vi "callC.vi"(8 "error in (no error)":errorcluster, 9 "constant command line":T1={"Red ball"={"R max"=255, "R min"=91, "G max"=80, "B max"=130, "B min"=0, "G min"=0}, "Yellow ball"={"R max"=255, "R min"=170, "G max"=255, "B max"=175, "B min"=0, "G min"=176}, "White ball"={"R max"=255, "R min"=100, "G max"=255, "B max"=250, "B min"=150, "G min"=150}, "Blue BG"={"R max"=62, "R min"=39, "G max"=116, "B max"=255, "B min"=202, "G min"=91}, "Ball diameter"=13}, 10 "billard rect":T2, 11 "Array":u32[][](array[numeric])) -> (0 "error out":errorcluster, 1 "White":cluster{"X":string, "Y":string}, 2 "Yellow":cluster{"X":string, "Y":string}, 3 "Red":cluster{"X":string, "Y":string}, 4 "standard error":string, 5 "standard output":string)   [LabVIEW 2021]
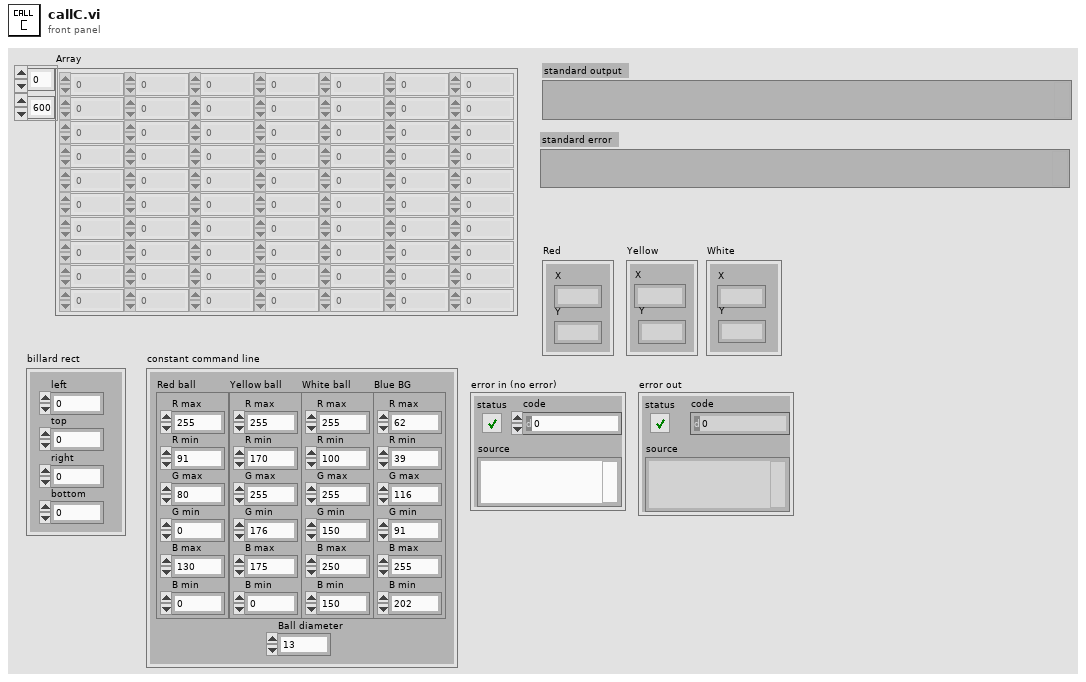
[diagram p1: front panel]
types:
  T1 = cluster{"Red ball":cluster{"R max":u8, "R min":u8, "G max":u8, "B max":u8, "B min":u8, "G min":u8}, "Yellow ball":cluster{"R max":u8, "R min":u8, "G max":u8, "B max":u8, "B min":u8, "G min":u8}, "White ball":cluster{"R max":u8, "R min":u8, "G max":u8, "B max":u8, "B min":u8, "G min":u8}, "Blue BG":cluster{"R max":u8, "R min":u8, "G max":u8, "B max":u8, "B min":u8, "G min":u8}, "Ball diameter":i32}
  T2 = cluster{"left":i32, "top":i32, "right":i32, "bottom":i32}
  T3 = enum16{"open", "replace", "create", "open or create", "replace or create", "replace or create with confirmation"}
  T4 = enum16{"big-endian, network order", "native, host order", "little-endian"}
  T5 = cluster{"result string":string, "result string":string}
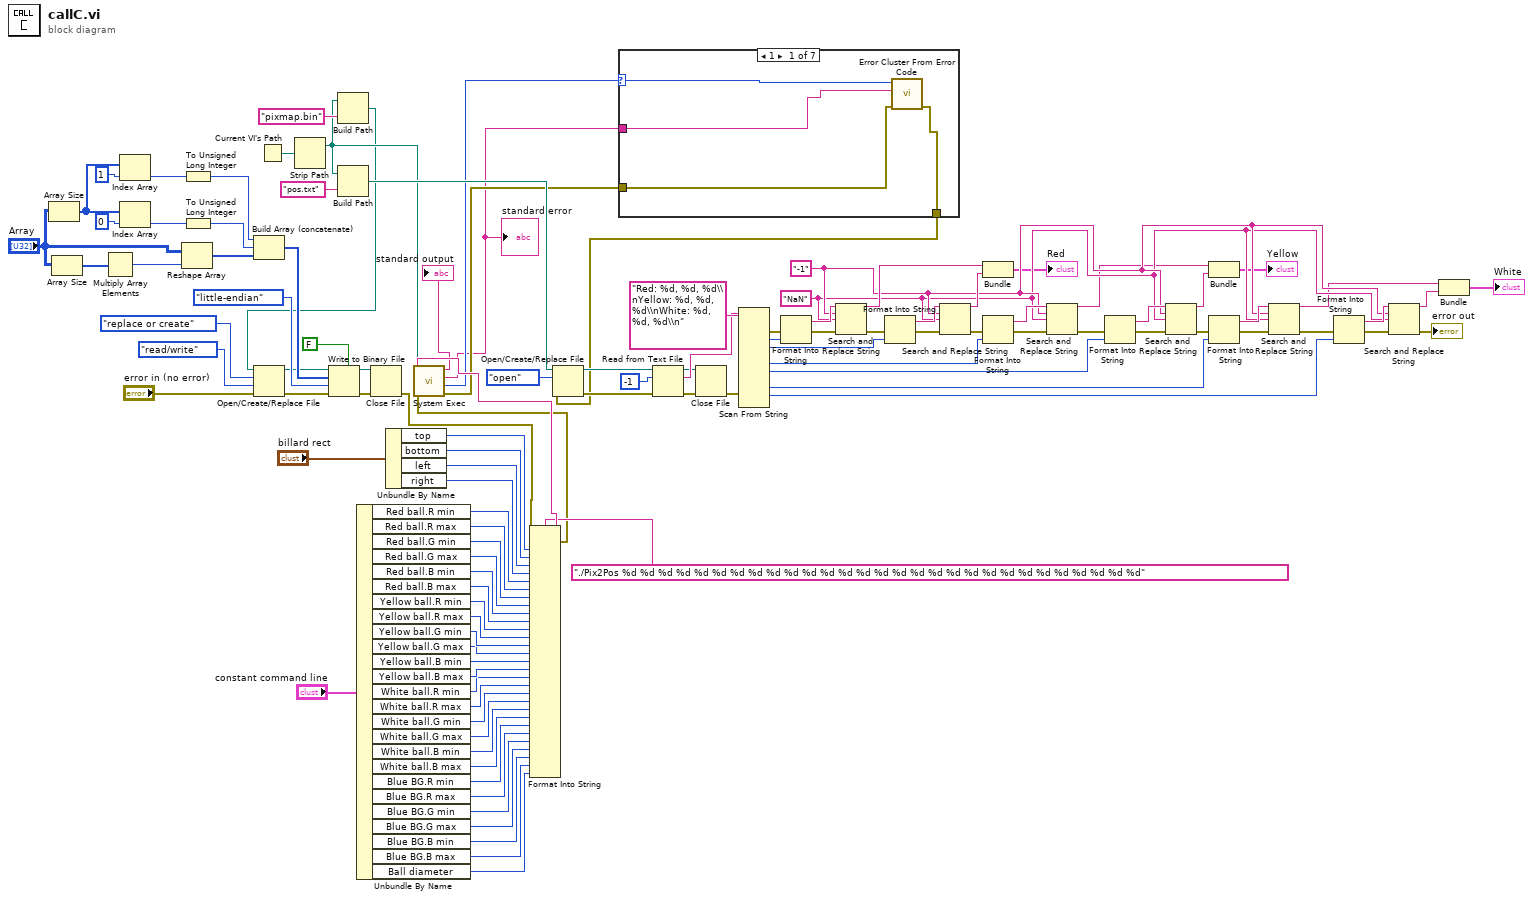
[diagram p0: block diagram]
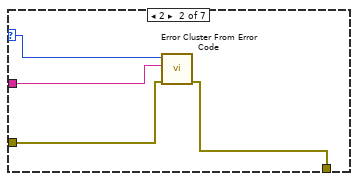
[diagram p2: hidden frame]
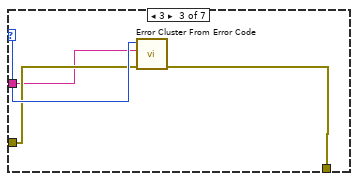
[diagram p3: hidden frame]
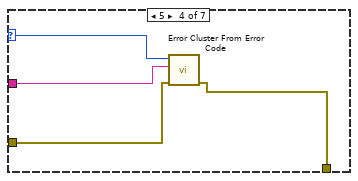
[diagram p4: hidden frame]
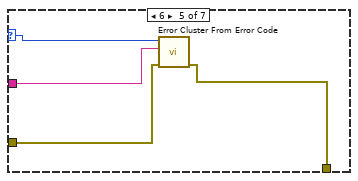
[diagram p5: hidden frame]
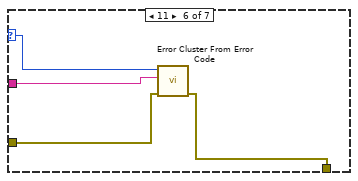
[diagram p6: hidden frame]
diagram:
  w72 = "NaN" ("replace string (\"\")")
  w73 = "-1" ("search string")
  n1 = Array Size(array="Array") -> (size(s)=w86:i32[])
  n2 = Array Size(array="Array") -> (size(s)=w84:i32[])
  n3 = Multiply Array Elements(1:w84) -> (0:w82:i32)
  n4 = Index Array(array=w86, index=1) -> (element=w109:i32)
  n5 = Index Array(array=w86, index=0) -> (element=w107:i32)
  n6 = Reshape Array("Array", w82) -> (w83:u32[])
  n7 = To Unsigned Long Integer(number=w109) -> (unsigned 32bit integer=w110:u32)
  n8 = To Unsigned Long Integer(number=w107) -> (unsigned 32bit integer=w108:u32)
  n9 = Build Array (concatenate)(w110, w108, w83) -> (w90:u32[])
  n10 = Current VI's Path() -> (path=w92:path)
  n11 = Strip Path(path=w92) -> (stripped path=w64:path)  [unwired: 1 out]
  n12 = Build Path(base path=w64, name or relative path="pixmap.bin") -> (appended path=w63:path)
  n13 = Open/Create/Replace File(file path (use dialog)=w63, error in="error in (no error)", operation (0:open)=T3."replace or create", access (0:read/write)=enum16{"read/write", "read-only", "write-only"}."read/write") -> (refnum out=w62:refnum<file>, error out=w60:errorcluster)  [unwired: 2 in, 1 out]
  n14 = Write to Binary File(file (use dialog)=w62, data=w90, error in=w60, 5:FALSE ("prepend array or string size? (T)"), 9:T4."little-endian" ("byte order (0:big-endian, network order)")) -> (refnum out=w58:refnum<file>, error out=w59:errorcluster)  [unwired: 1 in, 1 out]
  n15 = Build Path(base path=w64, name or relative path="pos.txt") -> (appended path=w104:path)
  n16 = Unbundle By Name("constant command line") -> ("Red ball.R min"=w54:u8, "Red ball.R max"=w53:u8, "Red ball.G min"=w52:u8, "Red ball.G max"=w51:u8, "Red ball.B min"=w50:u8, "Red ball.B max"=w49:u8, "Yellow ball.R min"=w48:u8, "Yellow ball.R max"=w47:u8, "Yellow ball.G min"=w46:u8, "Yellow ball.G max"=w45:u8, "Yellow ball.B min"=w44:u8, "Yellow ball.B max"=w43:u8, "White ball.R min"=w42:u8, "White ball.R max"=w41:u8, "White ball.G min"=w40:u8, "White ball.G max"=w39:u8, "White ball.B min"=w38:u8, "White ball.B max"=w37:u8, "Blue BG.R min"=w36:u8, "Blue BG.R max"=w35:u8, "Blue BG.G min"=w34:u8, "Blue BG.G max"=w33:u8, "Blue BG.B min"=w32:u8, "Blue BG.B max"=w31:u8, "Ball diameter"=w30:i32)
  n17 = Close File(refnum=w58, error in=w59) -> (error out=w19:errorcluster)  [unwired: 1 out]
  n18 = Unbundle By Name("billard rect") -> ("top"=w29:i32, "bottom"=w28:i32, "left"=w27:i32, "right"=w26:i32)
  n19 = Format Into String(format string="./Pix2Pos %d %d %d %d %d %d %d %d %d %d %d %d %d %d %d %d %d %d %d %d %d %d %d %d %d %d %d %d %d" ("command line"), error in=w19, w29, w28, w27, w26, w54, w53, w52, w51, w50, w49, w48, w47, w46, w45, w44, w43, w42, w41, w40, w39, w38, w37, w36, w35, w34, w33, w32, w31, w30) -> (resulting string=w106:string, error out=w18:errorcluster)  [unwired: 1 in]
  n20 = call <vilib>:"System Exec.vi"("error in (no error)"=w18, "working directory"=w64, "command line"=w106) -> ("error out"=w3:errorcluster, "return code"=w4:i32, "standard error"=w1:string, "standard output"=→"standard output":string)  [unwired: 5 in]
  "standard error" <- w1
  n21 = case shown="1" w4 {
    selector: w4 -> [w116 w120 w124 w128 w132 w136 _]
    tunnel: w3 -> [w115 w118 w123 w127 w130 w134 w137]
    tunnel: [w114 w117 w122 w126 w129 w133 w137] -> w2
    tunnel: w1 -> [w113 w119 w121 w125 w131 w135 _]
    frame 1 {
      n22 = call <vilib>:"Error Cluster From Error Code.vi"("error in (no error)"=w115, "error message (\"\")"=w113, "error code (0)"=w116) -> ("error out"=w114:errorcluster)  [unwired: 6 in]
    }
    frame 2 {
      n23 = call <vilib>:"Error Cluster From Error Code.vi"("error in (no error)"=w118, "error message (\"\")"=w119, "error code (0)"=w120) -> ("error out"=w117:errorcluster)  [unwired: 6 in]
    }
    frame 3 {
      n24 = call <vilib>:"Error Cluster From Error Code.vi"("error in (no error)"=w123, "error message (\"\")"=w121, "error code (0)"=w124) -> ("error out"=w122:errorcluster)  [unwired: 6 in]
    }
    frame 5 {
      n25 = call <vilib>:"Error Cluster From Error Code.vi"("error in (no error)"=w127, "error message (\"\")"=w125, "error code (0)"=w128) -> ("error out"=w126:errorcluster)  [unwired: 6 in]
    }
    frame 6 {
      n26 = call <vilib>:"Error Cluster From Error Code.vi"("error in (no error)"=w130, "error message (\"\")"=w131, "error code (0)"=w132) -> ("error out"=w129:errorcluster)  [unwired: 6 in]
    }
    frame 11 {
      n27 = call <vilib>:"Error Cluster From Error Code.vi"("error in (no error)"=w134, "error message (\"\")"=w135, "error code (0)"=w136) -> ("error out"=w133:errorcluster)  [unwired: 6 in]
    }
    frame Default {
    }
  }
  n28 = Open/Create/Replace File(file path (use dialog)=w104, error in=w2, operation (0:open)=T3."open") -> (refnum out=w98:refnum<file>, error out=w95:errorcluster)  [unwired: 3 in, 1 out]
  n29 = Read from Text File(file (use dialog)=w98, count=-1, error in=w95) -> (refnum out=w99:refnum<file>, text=w101:string, error out=w96:errorcluster)  [unwired: 1 in, 1 out]
  n30 = Close File(refnum=w99, error in=w96) -> (error out=w102:errorcluster)  [unwired: 1 out]
  n31 = Scan From String(format string="Red: %d, %d, %d\\nYellow: %d, %d, %d\\nWhite: %d, %d, %d\\n", input string=w101, error in=w102) -> (error out=w17:errorcluster, output 1=w25:i32, output 2=w24:i32, output 4=w23:i32, output 5=w22:i32, output 7=w21:i32, output 8=w20:i32)  [unwired: 13 in, 2 out]
  n32 = Format Into String(error in=w17, w25) -> (resulting string=w81:string, error out=w16:errorcluster)  [unwired: 2 in]
  n33 = Search and Replace String(input string=w81, search string=w73, replace string=w72, error in=w16) -> (result string=w80:string, error out=w15:errorcluster)  [unwired: 4 in, 2 out]
  n34 = Format Into String(error in=w15, w24) -> (resulting string=w79:string, error out=w14:errorcluster)  [unwired: 2 in]
  n35 = Search and Replace String(input string=w79, search string=w73, replace string=w72, error in=w14) -> (result string=w78:string, error out=w13:errorcluster)  [unwired: 4 in, 2 out]
  n36 = Bundle("result string"=w80, "result string"=w78) -> (→"Red":T5)  [unwired: 1 in]
  n37 = Format Into String(error in=w13, w23) -> (resulting string=w77:string, error out=w12:errorcluster)  [unwired: 2 in]
  n38 = Search and Replace String(input string=w77, search string=w73, replace string=w72, error in=w12) -> (result string=w71:string, error out=w11:errorcluster)  [unwired: 4 in, 2 out]
  n39 = Format Into String(error in=w11, w22) -> (resulting string=w76:string, error out=w10:errorcluster)  [unwired: 2 in]
  n40 = Search and Replace String(input string=w76, search string=w73, replace string=w72, error in=w10) -> (result string=w70:string, error out=w9:errorcluster)  [unwired: 4 in, 2 out]
  n41 = Bundle("result string"=w71, "result string"=w70) -> (→"Yellow":T5)  [unwired: 1 in]
  n42 = Format Into String(error in=w9, w21) -> (resulting string=w75:string, error out=w8:errorcluster)  [unwired: 2 in]
  n43 = Search and Replace String(input string=w75, search string=w73, replace string=w72, error in=w8) -> (result string=w69:string, error out=w7:errorcluster)  [unwired: 4 in, 2 out]
  n44 = Format Into String(error in=w7, w20) -> (resulting string=w74:string, error out=w6:errorcluster)  [unwired: 2 in]
  n45 = Search and Replace String(input string=w74, search string=w73, replace string=w72, error in=w6) -> (result string=w68:string, error out=→"error out":errorcluster)  [unwired: 4 in, 2 out]
  n46 = Bundle("result string"=w69, "result string"=w68) -> (→"White":T5)  [unwired: 1 in]
